vi "Rollers.vi"(11 "Roller Command":T2) -> (0 "Halo":bool, 1 "Back Motor":dbl, 2 "Front Solenoid":T1, 3 "Front Motor":dbl, 4 "Net Solenoid":T1)   [LabVIEW 2013]
uses:
  Roller Control.ctl
  Roller Mode.ctl
  <vilib>/Rock Robotics/WPI/Solenoid/WPI_SolenoidValue.ctl
  Robot Global Data.vi
panel:
  in  "Roller Speed Back":dbl
  in  "Roller Speed Front":dbl
  # "Debug controls under this box"
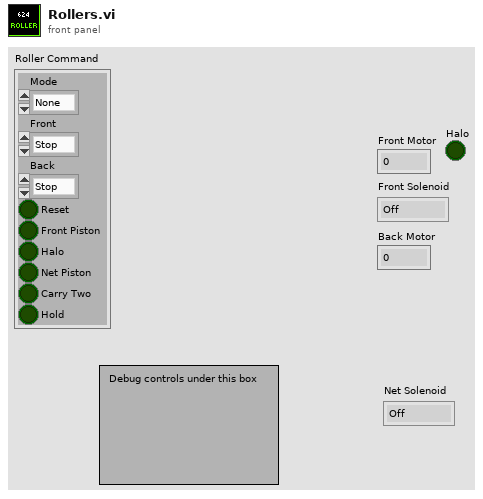
[diagram p1: front panel]
types:
  T1 = typedef "WPI_SolenoidValue.ctl" = enum16{"Off", "On", "Forward", "Reverse"}
  T2 = typedef "Roller Control.ctl" = cluster{"Mode":T3, "Front":enum16{"Stop", "Forward", "Reverse"}, "Back":enum16{"Stop", "Forward", "Reverse"}, "Reset":bool, "Front Piston":bool, "Halo":bool, "Net Piston":bool, "Carry Two":bool, "Hold":bool}
  T3 = typedef "Roller Mode.ctl" = enum16{"None", "Front", "Back", "Both", "Manual"}
  T4 = typedef "Dashboard UDP Packet.ctl" = cluster{"Camera":T5, "Gyro":T6, "Encoder":T8, "Auto Shift":T9, "Auton":T10, "Drive/Ramp X":dbl, "Drive/Ramp Y":dbl, "Drive/Battery Cutoff":dbl, "Pressure/Compressor Min Voltage":dbl, "Pressure/Compressor Delay":dbl, "Controller/Strafe Correction":bool, "Shooter":T11, "Rollers":T12, "Abort":bool, "Finish":bool, "Shooter Halo Time":dbl, "IR Halo Sustain Time":dbl, "Disable Compressor":bool}
  T5 = typedef "Camera Controls.ctl" = cluster{"Camera/View Angle X":dbl, "Camera/Goal Track Timeout":dbl, "Camera/View Angle Y":dbl, "Camera/Goal Exposure":dbl, "Camera/Vision Receive Timeout":dbl, "Camera/Offset 1":dbl, "Camera/Offset 2":dbl}
  T6 = typedef "Gyro Controls.ctl" = cluster{"Gyro/Angle Tolerance":dbl, "Gyro/Steer Closeness Threshold":dbl, "Steer PID":T7, "Steer Close PID":T7}
  T7 = typedef "PID Params.ctl" = cluster{"max":dbl, "min":dbl, "P":dbl, "I":dbl, "D":dbl}
  T8 = typedef "Encoder Controls.ctl" = cluster{"Encoders/Reset":bool, "Encoders/Omni Constant":dbl, "Encoders/Omni Tick Constant":dbl, "Encoders/Left Constant":dbl, "Encoders/Right Constant":dbl, "Encoders/Right Tick Constant":dbl}
  T9 = typedef "Auto Shift Controls.ctl" = cluster{"AutoShift/Upshift Throttle Accel":dbl, "AutoShift/Speed Threshold":dbl, "AutoShift/Upshift Throttle":dbl, "AutoShift/Upshift Accel":dbl, "AutoShift/Downshift Accel":dbl, "AutoShift/Downshift Throttle":dbl, "AutoShift/Delay":dbl, "AutoShift/Enabled":bool}
  T10 = typedef "Auton Controls.ctl" = cluster{"Auton/Left Shoot X-Coord":dbl, "Auton/Right Shoot X-Coord":dbl, "DistDrive/Distance Stop Threshold":dbl, "DistDrive/Max Stop Speed":dbl, "Auton/Back Piston Time":dbl, "Auton/Manual Hot":bool, "Auton/Manual Hot Right":bool, "Default X PID":T7, "Default Y PID":T7}
  T11 = typedef "Shooter Controls.ctl" = cluster{"Shooter/Reset Time":dbl, "Shooter/Release Delay":dbl, "Shooter/Pressure Steady Time":dbl, "Shooter/Misfire Delay":dbl, "Shooter/Ball Settle Time":dbl, "Shooter/Line IR Delay":dbl, "Pressure/Upper PSI Time":dbl, "Pressure/Lower PSI Time":dbl, "Shooter/Punch Delay":dbl, "Shooter/Target Pressure":dbl, "Pressure/Line B":dbl, "Pressure/Line M":dbl, "Pressure/Shooter M":dbl, "Pressure/Shooter B":dbl}
  T12 = typedef "Roller Controls.ctl" = cluster{"Roller/Load IRs Verify Time":dbl, "Roller/Center IR Latch Time":dbl, "Roller/Speed Front":dbl, "Roller/Speed Back":dbl, "Roller/Entry Timeout":dbl, "Roller/To Center Timeout":dbl, "Roller/Sustain Time":dbl, "Roller/Verify Center Time":dbl}
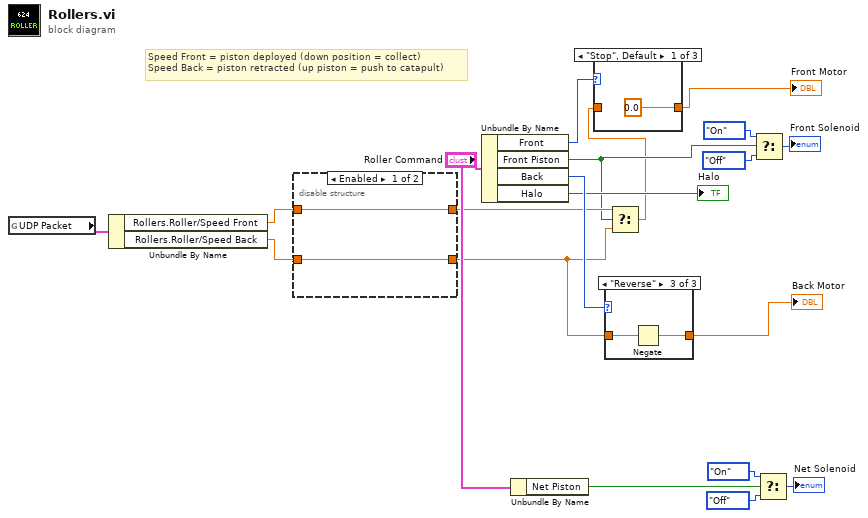
[diagram p0: block diagram]
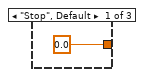
[diagram p2: hidden frame]
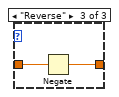
[diagram p5: hidden frame]
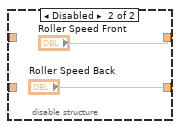
[diagram p6: hidden frame]
diagram:
  # "Speed Front = piston deployed (down position = collect)\nSpeed Back = piston retracted (up piston = push to catapult)"
  n1 = global read "Robot Global Data.vi" "UDP Packet"() -> (w8:T4)
  n2 = Unbundle By Name(w8) -> ("Rollers.Roller/Speed Front"=w7:dbl, "Rollers.Roller/Speed Back"=w6:dbl)
  n3 = disable-structure shown="Enabled" {
    disable-tunnel: [w22 "Roller Speed Front"] -> w4
    disable-tunnel: [w21 "Roller Speed Back"] -> w3
    disable-tunnel: w7 -> [w22 _]
    disable-tunnel: w6 -> [w21 _]
    frame Enabled {
    }
    frame Disabled {
    }
  }
  n4 = Unbundle By Name("Roller Command") -> ("Front"=w11:enum16{"Stop", "Forward", "Reverse"}, "Front Piston"=w2:bool, "Back"=w10:enum16{"Stop", "Forward", "Reverse"}, "Halo"=→"Halo":bool)
  n5 = Unbundle By Name("Roller Command") -> ("Net Piston"=w13:bool)
  n6 = case shown="\"Reverse\"" w10 {
    tunnel: [0.0 ("Roller Speed Front") w26 w27] -> w9
    tunnel: w3 -> [_ w26 w28]
    frame "Stop", Default {
    }
    frame "Forward" {
    }
    frame "Reverse" {
      n7 = Negate(x=w28) -> (-x=w27:dbl)
    }
  }
  "Back Motor" <- w9
  n8 = Select(t=w4, s=w2, f=w3) -> (s? t:f=w1:dbl)
  n9 = case shown="\"Stop\", Default" w11 {
    tunnel: [0.0 ("Roller Speed Front") w30 w31] -> w12
    tunnel: w1 -> [_ w30 w32]
    frame "Stop", Default {
    }
    frame "Forward" {
    }
    frame "Reverse" {
      n10 = Negate(x=w32) -> (-x=w31:dbl)
    }
  }
  "Front Motor" <- w12
  n11 = Select(t=WPI_SolenoidValue."On" ("Solenoid Output"), s=w2, f=WPI_SolenoidValue."Off" ("Solenoid Output")) -> (s? t:f=→"Front Solenoid":T1)
  n12 = Select(t=WPI_SolenoidValue."On" ("Solenoid Output"), s=w13, f=WPI_SolenoidValue."Off" ("Solenoid Output")) -> (s? t:f=→"Net Solenoid":T1)
